vi "Ensure Dependencies Started.vi"(8 "error in (no error)":errorcluster, 10 "Dependency in":refnum<class "SMO.lvclass">, 11 "SMO in":refnum<class "SMO.lvclass">) -> (0 "error out":errorcluster, 2 "Started Dependency":refnum<class "SMO.lvclass">, 3 "SMO out":refnum<class "SMO.lvclass">)   [LabVIEW 2013, in "SMO.lvclass"]
uses:
  SMO.lvclass
  SMO.lvclass/SMO.ctl
  Support/Attribute.Owner/Attribute.Owner.lvclass/Attribute.Owner.ctl
  Typedefs/SMO Dependency Event--Cluster.ctl
  Typedefs/SMO Dependency Event--Enum.ctl
  Support/Attribute.Identity/Attribute.Identity.lvclass/Attribute.Identity.ctl
  ReftoDVR--SMO.vi
  Support/Attribute.Owner/Verify Key Match.vi
  GetVariant(Attr).vi
  Support/Attribute.Identity/Read UniqueName.vi
  Support/Attribute.Identity/Read Given Name.vi
  Support/Attribute.Identity/Read ProspectiveOwner.vi
  Support/Attribute.Owner/Read Shared Key.vi
  <vilib>/Utility/MD5Checksum.llb/MD5Checksum string.vi
  Support/Attribute.Owner/Attribute.Owner.lvclass
  Support/Attribute.Identity/Attribute.Identity.lvclass
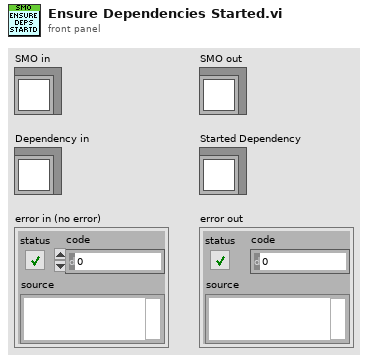
[diagram p1: front panel]
types:
  T1 = typedef "SMO.lvclass/SMOState --Enum.ctl" = enum16{"unknown", "Created", "Started", "Stopped"}
  T2 = typedef "SMO.lvclass/Protected Events.ctl" = cluster{"StopProcesses":refnum<user-event>, "AbortProcesses":refnum<user-event>, "Config Changed":refnum<user-event>, "Dependency":refnum<user-event>}
  T3 = typedef "SMO.lvclass/SMO Dependency Event--Enum.ctl" = enum16{"Added", "Removed", "Started", "Stopped"}
  T4 = typedef "SMO.lvclass/SMO Dependency Event--Cluster.ctl" = cluster{"Name":string, "GUID":string, "Event":T3}
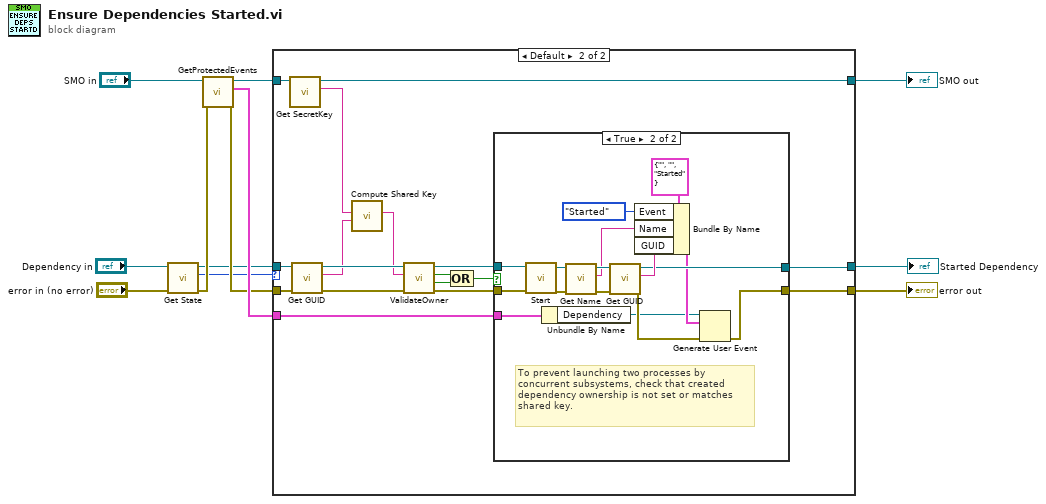
[diagram p0: block diagram]
diagram:
  n1 = call "Get State.vi"("error in (no error)"="error in (no error)", "SMO"="Dependency in") -> ("error out"=w8:errorcluster, "SMO State"=w6:T1, "SMO out"=w4:refnum<class "SMO.lvclass">)  [unwired: 7 in]
  n2 = call "GetProtectedEvents.vi"("error in (no error)"=w8, "SMO"="SMO in") -> ("error out"=w9:errorcluster, "SMO Protected Events"=w10:T2, "SMO out"=w2:refnum<class "SMO.lvclass">)  [unwired: 7 in]
  n3 = case shown="Default" w6 {
    tunnel: [w14 w31] -> w3
    tunnel: [w15 w32] -> w7
    tunnel: w4 -> [w15 w20]
    tunnel: w9 -> [w14 w22]
    tunnel: w10 -> [_ w30]
    tunnel: w2 -> [w13 w24]
    tunnel: [w13 w23] -> w1
    frame "Started" {
    }
    frame Default {
      n4 = call "Get SecretKey.vi"("SMO"=w24) -> ("SecretKey"=w18:string, "SMO out"=w23:refnum<class "SMO.lvclass">)  [unwired: 8 in, 1 out]
      n5 = call "Get GUID.vi"("error in (no error)"=w22, "SMO"=w20) -> ("error out"=w21:errorcluster, "GUID"=w17:string, "SMO out"=w19:refnum<class "SMO.lvclass">)  [unwired: 7 in]
      n6 = call "Compute Shared Key.vi"("GUID"=w17, "SecretKey"=w18) -> ("Shared Key"=w16:string)  [unwired: 9 in]
      n7 = call "ValidateOwner.vi"("error in (no error)"=w21, "Shared Key"=w16, "SMO in"=w19) -> ("error out"=w29:errorcluster, "not set"=w26:bool, "key matched"=w27:bool, "SMO out"=w28:refnum<class "SMO.lvclass">)  [unwired: 5 in]
      n8 = Compound Arithmetic op=OR(w27, w26) -> (w25:bool)
      n9 = case shown="True" w25 {
        tunnel: [w34 w43] -> w32
        tunnel: [w33 w40] -> w31
        tunnel: w30 -> [_ w38]
        tunnel: w29 -> [w33 w36]
        tunnel: w28 -> [w34 w35]
        frame False {
        }
        frame True {
          # "To prevent launching two processes by\nconcurrent subsystems, check that created\ndependency ownership is not set or matches\nshared key."
          n10 = call "Start.vi"("error in (no error)"=w36, "SMO"=w35) -> ("error out"=w47:errorcluster, "SMO out"=w48:refnum<class "SMO.lvclass">)  [unwired: 8 in]
          n11 = Unbundle By Name(w38) -> ("Dependency"=w39:refnum<user-event>)
          n12 = call "Get Name.vi"("error in (no error)"=w47, "SMO"=w48) -> ("error out"=w50:errorcluster, "Name"=w45:string, "SMO out"=w49:refnum<class "SMO.lvclass">)  [unwired: 5 in, 2 out]
          n13 = call "Get GUID.vi"("error in (no error)"=w50, "SMO"=w49) -> ("error out"=w41:errorcluster, "GUID"=w44:string, "SMO out"=w43:refnum<class "SMO.lvclass">)  [unwired: 7 in]
          n14 = Bundle By Name(cluster=T4 {"Name"="", "GUID"="", "Event"=enum."Started"} ("Dependency Event"), "Event"=SMO_Dependency_Event--Enum."Started", "Name"=w45, "GUID"=w44) -> (w42:T4)
          n15 = Generate User Event(user event=w39, event data cluster=w42, error in=w41) -> (error out=w40:errorcluster)  [unwired: 1 in, 1 out]
        }
      }
    }
  }
  "SMO out" <- w1
  "Started Dependency" <- w7
  "error out" <- w3
